vi "SingleJointedArmSim_example.vi"() -> ()   [LabVIEW 2019]
uses:
  <vilib>/Rock Robotics/WPI/ThirdParty/JAS_Junk/TrajLib/DCMOTOR.CTL
  <vilib>/Rock Robotics/WPI/ThirdParty/JAS_Junk/TrajLib/LINEAR_SYSTEM.ctl
  <vilib>/Analysis/Matrix/Datatypes/RealMatrix.ctl
  <vilib>/Rock Robotics/WPI/ThirdParty/JAS_Junk/TrajLib/LINEAR_QUADRATIC_REGULATOR.ctl
  <vilib>/Rock Robotics/WPI/ThirdParty/JAS_Junk/TrajLib/KALMAN_FILTER.ctl
  <vilib>/Rock Robotics/WPI/ThirdParty/JAS_Junk/TrajLib/LINEAR_SYSTEM_LOOP.ctl
  <vilib>/Rock Robotics/WPI/ThirdParty/JAS_Junk/TrajLib/LINEAR_PLANT_INV_FF.ctl
  <vilib>/Rock Robotics/WPI/ThirdParty/JAS_Junk/TrajLib/SINGLE_JOINT_ARM_SIM.ctl
  <vilib>/Rock Robotics/WPI/ThirdParty/JAS_Junk/TrajLib/LINEAR_SYSTEM_SIM.ctl
  <vilib>/Rock Robotics/WPI/ThirdParty/JAS_Junk/TrajLib/MatBuilder_Create.vi
  <vilib>/Rock Robotics/WPI/ThirdParty/JAS_Junk/TrajLib/DCMotor_New.vi
  <vilib>/Rock Robotics/WPI/ThirdParty/JAS_Junk/TrajLib/Units_RotationsPerMinuteToRadiansPerSecond.vi
  <vilib>/Rock Robotics/WPI/ThirdParty/JAS_Junk/TrajLib/LinearSystem_New.vi
  <vilib>/Rock Robotics/WPI/ThirdParty/JAS_Junk/TrajLib/MatrixHelper_Zero.vi
  <vilib>/Rock Robotics/WPI/ThirdParty/JAS_Junk/TrajLib/MatBuilder_Fill.vi
  <vilib>/Rock Robotics/WPI/ThirdParty/JAS_Junk/TrajLib/MatrixHelper_CoerceSize.vi
  <vilib>/Rock Robotics/WPI/ThirdParty/JAS_Junk/TrajLib/Trajectory_Library.lvlib
  <vilib>/Analysis/Matrix/NI_Matrix.lvlib
panel:
  in  "Tab Control":T1(tab)
  out "Battery Voltage":dbl format="%20.3f"
  out "CO Chart":cluster{dbl, "Voltage":dbl}(graph)
  in  "Move Arm":bool
  out "Arm Position\nRadians":dbl(slide) scale=-1.0..4.0
  out "Arm Angle":dbl format="%20.3f"
  out "Cor Err":bool
  out "Kalman Filtered\nArm Angle":dbl format="%20.3f"
  out "PV Chart":T2(graph)
  out "Predict Err":bool
  out "Motor Volt Dmd (CO)":dbl format="%20.3f"
  out "At Top":bool
  out "At Bottom":bool
  out "Motor Amps":dbl format="%20.3f"
  out "Arm Motor":T3 {"Jr_KgM2" format="%13.5p"; "L_H" format="%13.5p"; "Kt_NMPerAmp" format="%13.5p"; "KvINV_RadPerSecPerVolt" format="%13.5p"; "R_Ohms" format="%13.5p"; "FreeSpeed_RadPerSec" format="%13.5p"; "FreeCurrent_Amps" format="%13.5p"; "StallCurrent_Amps" format="%13.5p"; "StallTorque_NM" format="%13.5p"; "nominalVoltage_Volts" format="%13.5p"}
  out "m_Arm":T4
  out "Single Joint Arm Simulaation":T6 {"GearBox"."Jr_KgM2" format="%13.5p"; "GearBox"."L_H" format="%13.5p"; "GearBox"."Kt_NMPerAmp" format="%13.5p"; "GearBox"."KvINV_RadPerSecPerVolt" format="%13.5p"; "GearBox"."R_Ohms" format="%13.5p"; "GearBox"."FreeSpeed_RadPerSec" format="%13.5p"; "GearBox"."FreeCurrent_Amps" format="%13.5p"; "GearBox"."StallCurrent_Amps" format="%13.5p"; "GearBox"."StallTorque_NM" format="%13.5p"; "GearBox"."nominalVoltage_Volts" format="%13.5p"}
  out "KalmanFilter":T8
  out "Kalman Error":errorcluster
  out "LinearQuadraticRegulator":T9
  out "LQR Error":bool
  out "Linear System Loop":T10
  out "LinSysLoop_Error":bool
  # "<States,States>"
  # "<States,Inputs>"
  # "<Outputs,States>"
  # "<Outputs,Inputs>"
  # "<States, 1>"
  # "<Outputs, 1>"
  # "<Inputs, 1>"
  # "<Outputs, 1>"
  # "<States,States>"
  # "<States,Inputs>"
  # "<Outputs,States>"
  # "<Outputs,Inputs>"
  # "Steady State Gain  \n<States,Outputs>"
  # "State Estimate <Statess,1>"
  # "<States,States>"
  # "<States,Inputs>"
  # "<Outputs,States>"
  # "<Outputs,Inputs>"
  # "Ref State <States,1>"
  # "Comp and capped \noutput <Inputs,1>"
  # "Controller gain\n<Inputs,States>"
  # "<States,1>"
  # "<FUTURE --- CLAMP TYPE -- For now\nuse Normalize>"
  # "Steady State Gain  \n<States,Outputs>"
  # "State Estimate <Statess,1>"
  # "<States,States>"
  # "<States,Inputs>"
  # "<Outputs,States>"
  # "<Outputs,Inputs>"
  # "<States,1>"
  # "<Inputs,1>"
  # "<States,Inputs>"
  # "<States,States>"
  # "Ref State <States,1>"
  # "Comp and capped \noutput <Inputs,1>"
  # "Controller gain\n<Inputs,States>"
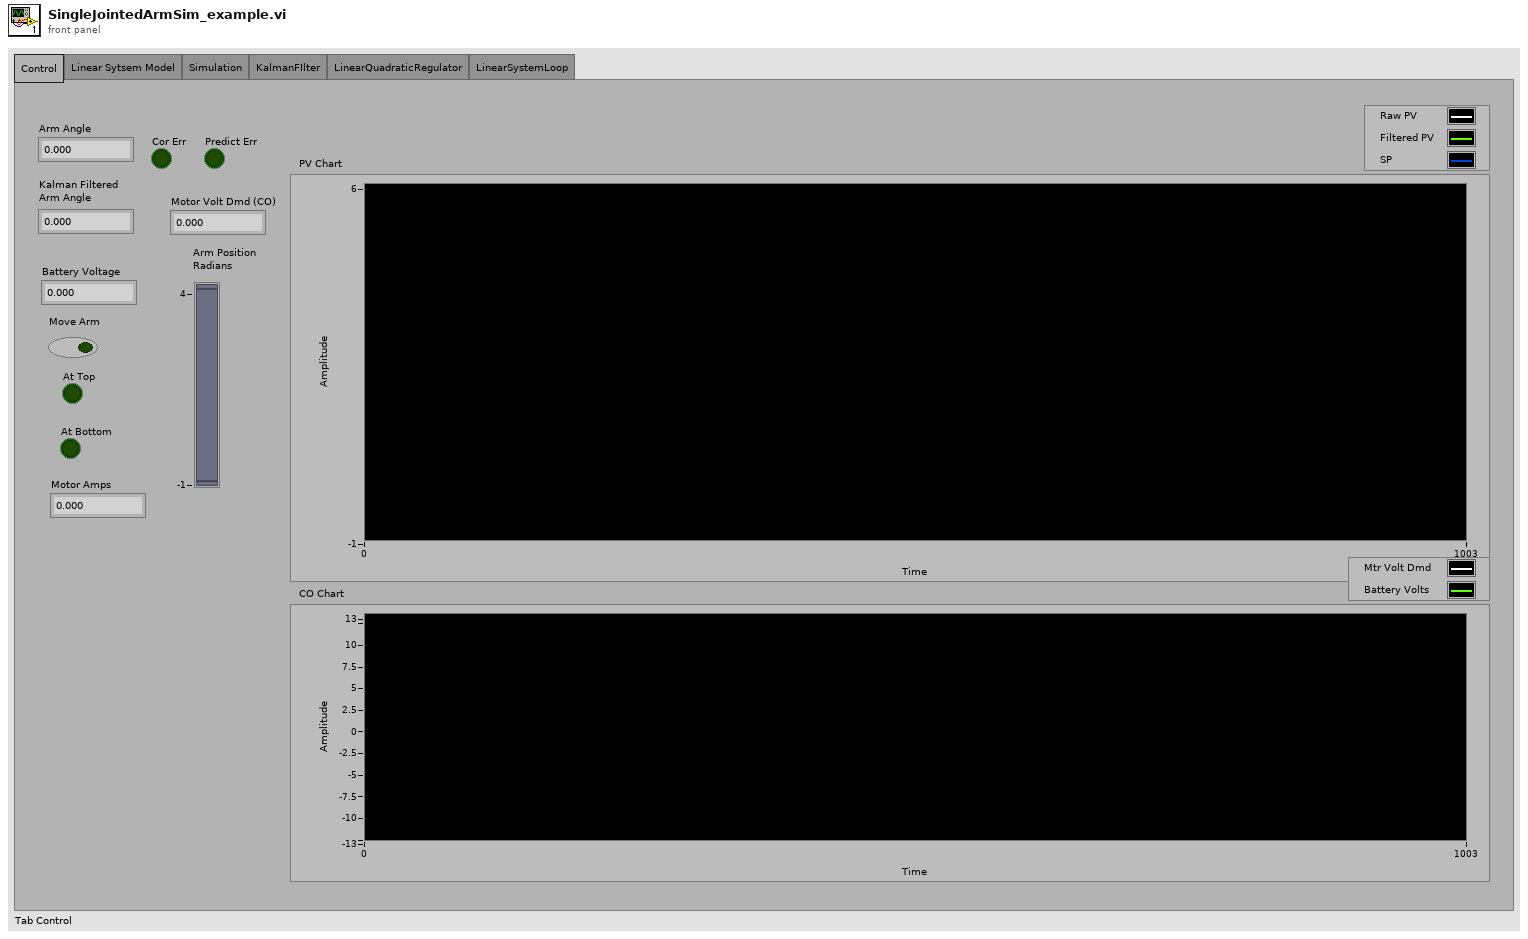
[diagram p1: front panel]
types:
  T1 = enum32{"Control", "Linear Sytsem Model", "Simulation", "KalmanFIlter", "LinearQuadraticRegulator", "LinearSystemLoop"}
  T2 = cluster{"upper limit":dbl, "Real Matrix Element":dbl, "Real Matrix Element":dbl}
  T3 = typedef "Trajectory_Library.lvlib/DCMOTOR.CTL" = cluster{"nominalVoltage_Volts":dbl, "StallTorque_NM":dbl, "StallCurrent_Amps":dbl, "FreeCurrent_Amps":dbl, "FreeSpeed_RadPerSec":dbl, "R_Ohms":dbl, "KvINV_RadPerSecPerVolt":dbl, "Kt_NMPerAmp":dbl, "L_H":dbl, "Jr_KgM2":dbl}
  T4 = typedef "Trajectory_Library.lvlib/LINEAR_SYSTEM.ctl" = cluster{"m_A":T5, "m_B":T5, "m_C":T5, "m_D":T5, "States":i32, "Inputs":i32, "Outputs":i32}
  T5 = typedef "NI_Matrix.lvlib/RealMatrix.ctl" = dbl[][]
  T6 = typedef "Trajectory_Library.lvlib/SINGLE_JOINT_ARM_SIM.ctl" = cluster{"Arm_LinearSystem":T7, "GearBox":T3, "Gearing":dbl, "R_ArmLength_M":dbl, "MinAngle_Rad":dbl, "MaxAngle_Rad":dbl, "ArmMass_Kg":dbl, "SimulateGravity":bool}
  T7 = typedef "Trajectory_Library.lvlib/LINEAR_SYSTEM_SIM.ctl" = cluster{"m_Plant":T4, "m_X":T5, "m_Y":T5, "m_U":T5, "MeasureStdDev":T5}
  T8 = typedef "Trajectory_Library.lvlib/KALMAN_FILTER.ctl" = cluster{"m_K":T5, "m_xHat":T5, "States":i32, "Outputs":i32, "m_Plant":T4}
  T9 = typedef "Trajectory_Library.lvlib/LINEAR_QUADRATIC_REGULATOR.ctl" = cluster{"m_r":T5, "m_U":T5, "m_K":T5, "States":i32, "Inputs":i32}
  T10 = typedef "Trajectory_Library.lvlib/LINEAR_SYSTEM_LOOP.ctl" = cluster{"Controller":T9, "FeedForward":T11, "Observer":T8, "Next_R":T5, "Clamp Max":T5}
  T11 = typedef "Trajectory_Library.lvlib/LINEAR_PLANT_INV_FF.ctl" = cluster{"m_R":T5, "m_Uff":T5, "m_B":T5, "m_A":T5, "States":i32, "Inputs":i32}
  T12 = cluster{"ArmAngle_Rad":dbl, "Real Matrix Element":dbl, "Real Matrix Element":dbl}
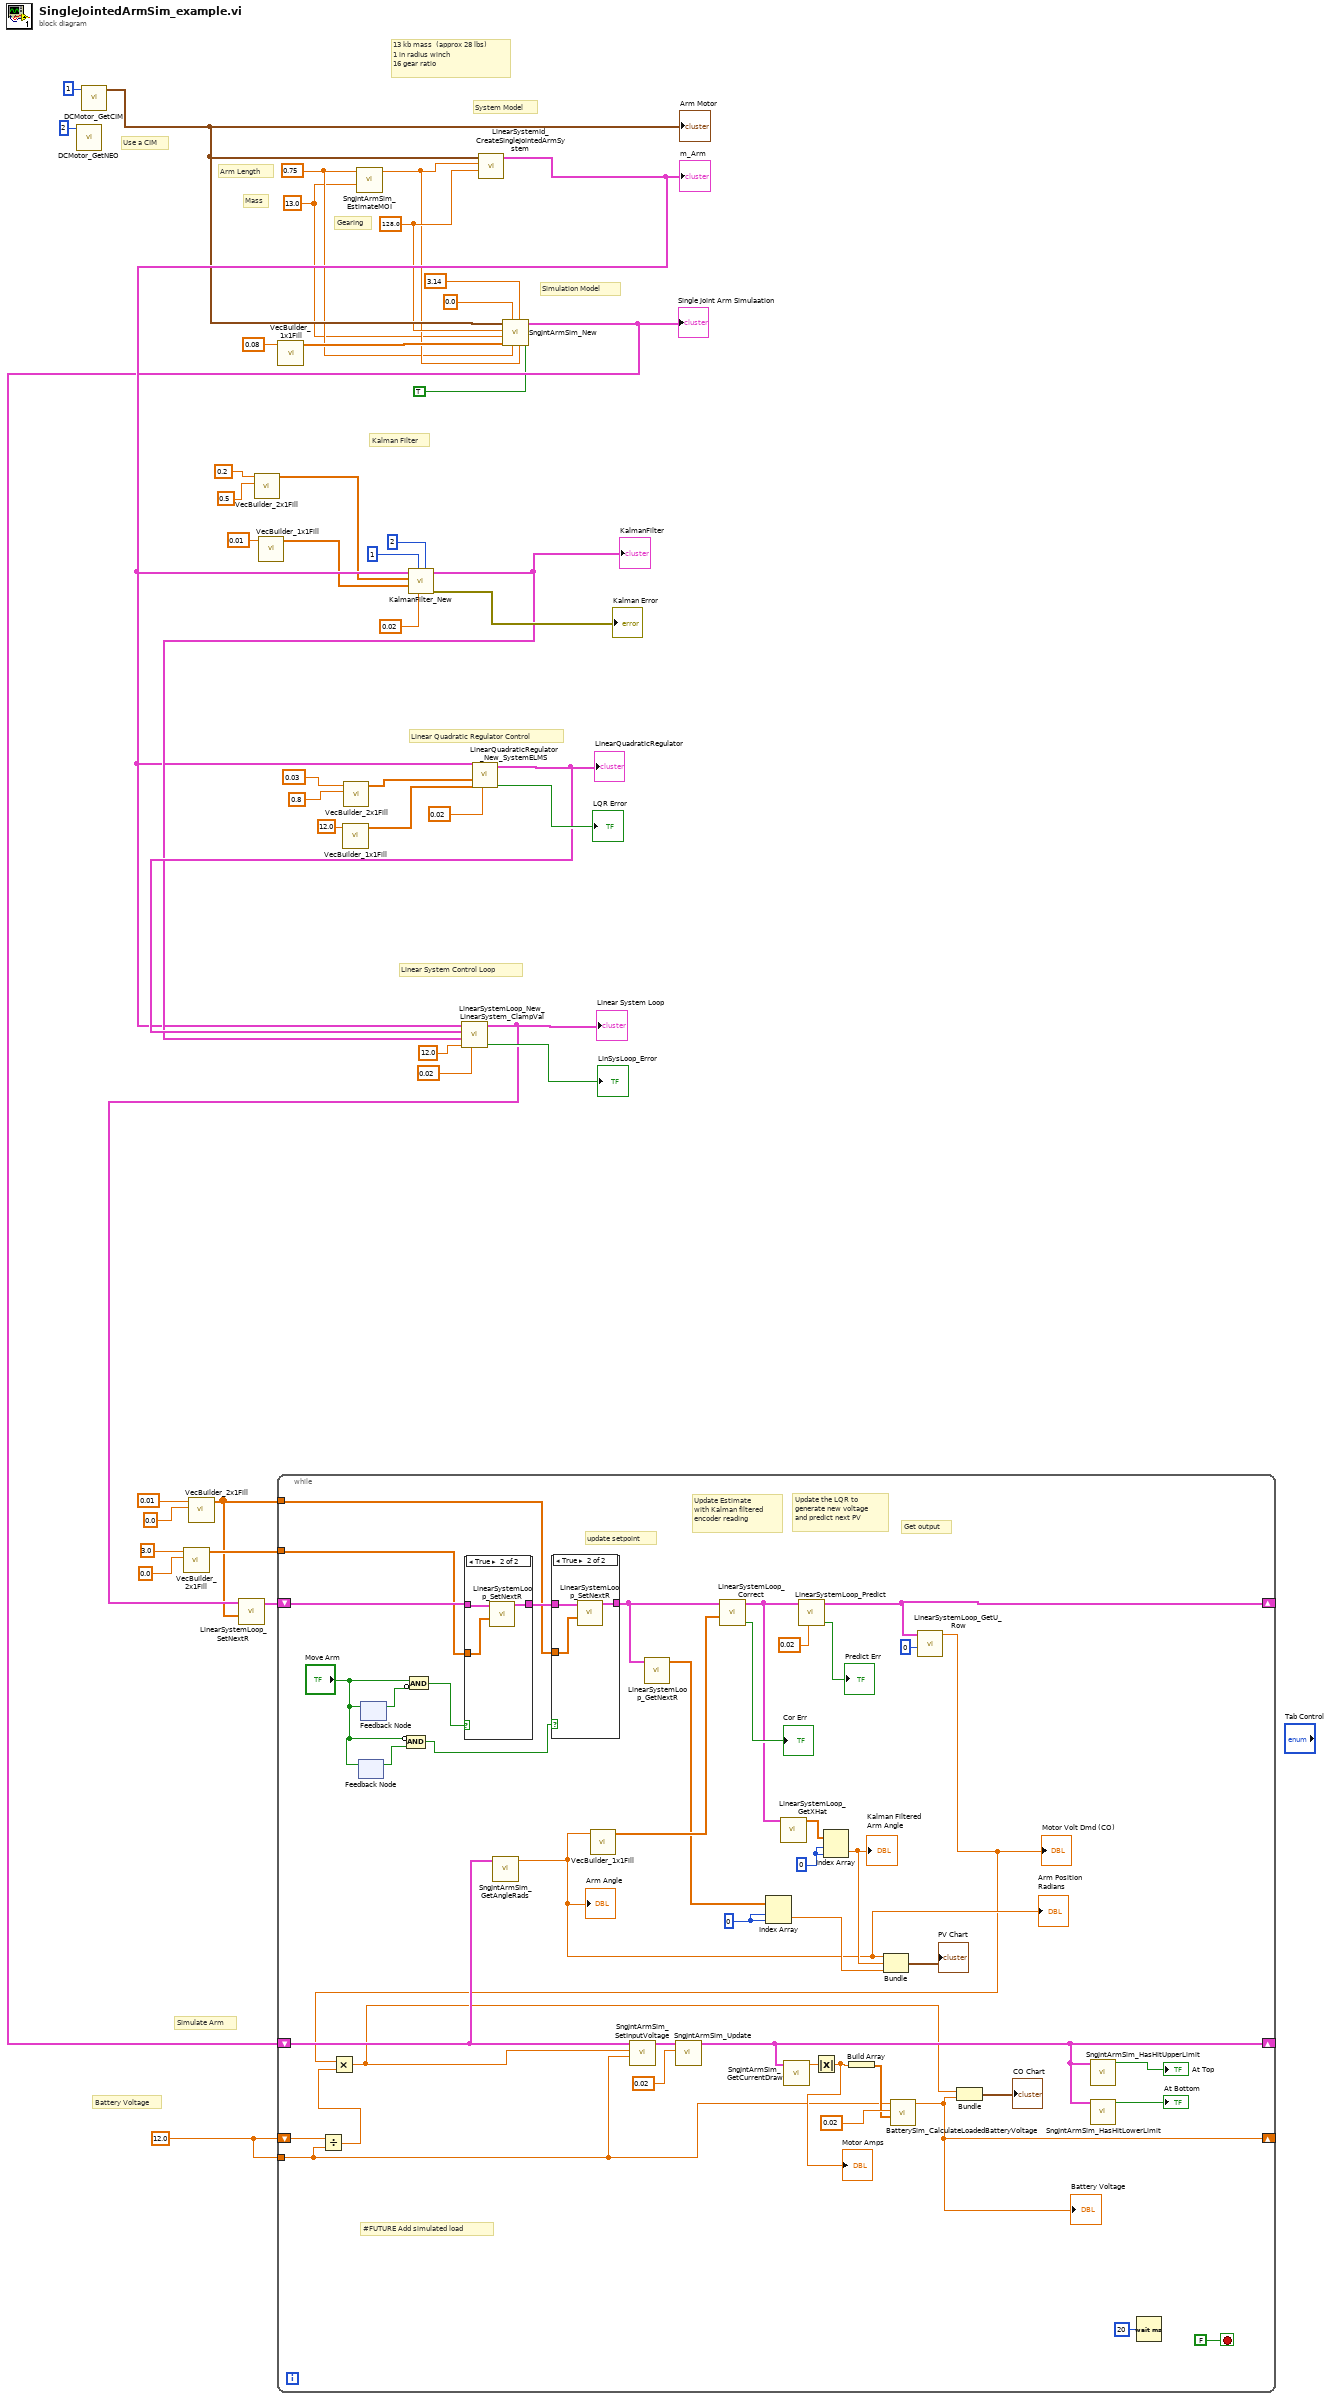
[diagram p0: block diagram]
diagram:
  w4 = 0.75 ("ArmLength_M")
  w7 = 128.0 ("G")
  w3 = 13.0 ("massKg")
  w36 = 12.0
  # "Simulation Model"
  # "System Model"
  # "Arm Length"
  # "Mass"
  # "Kalman Filter"
  # "Linear Quadratic Regulator Control"
  # "Linear System Control Loop"
  # "Simulate Arm"
  # "13 kb mass  (approx 28 lbs)\n1 in radius winch\n16 gear ratio"
  # "Gearing"
  # "Use a CIM"
  # "Battery Voltage"
  n1 = call <vilib>:"DCMotor_GetNEO.vi"("Num Motors"=2) -> ()  [unwired: 10 in, 1 out]
  n2 = call <vilib>:"DCMotor_GetCIM.vi"("Num Motors"=1) -> ("DCMOTOR"=w10:T3)  [unwired: 10 in]
  "Arm Motor" <- w10
  n3 = call <vilib>:"VecBuilder_2x1Fill.vi"("R1"=0.0, "R0"=3.0 ("RotationsPerMinute")) -> ("output matrix"=w16:T5)  [unwired: 9 in]
  n4 = call <vilib>:"VecBuilder_2x1Fill.vi"("R1"=0.0, "R0"=0.01 ("R0_C0")) -> ("output matrix"=w1:T5)  [unwired: 9 in]
  n5 = call <vilib>:"VecBuilder_2x1Fill.vi"("R1"=0.5, "R0"=0.2 ("R0_C0")) -> ("output matrix"=w27:T5)  [unwired: 9 in]
  n6 = call <vilib>:"VecBuilder_1x1Fill.vi"("R0_C0"=0.01) -> ("output matrix"=w26:T5)  [unwired: 10 in]
  n7 = call <vilib>:"VecBuilder_1x1Fill.vi"("R0_C0"=0.08) -> ("output matrix"=w6:T5)  [unwired: 10 in]
  n8 = call <vilib>:"VecBuilder_1x1Fill.vi"("R0_C0"=12.0) -> ("output matrix"=w20:T5)  [unwired: 10 in]
  n9 = call <vilib>:"VecBuilder_2x1Fill.vi"("R1"=0.8 ("R0_C0"), "R0"=0.03 ("R0_C0")) -> ("output matrix"=w22:T5)  [unwired: 9 in]
  n10 = call <vilib>:"SngJntArmSim_EstimateMOI.vi"("ArmMass_Kg"=w3, "ArmLength_M"=w4) -> ("MOI"=w5:dbl)  [unwired: 9 in]
  n11 = call <vilib>:"LinearSystemId_CreateSingleJointedArmSystem.vi"("G"=w7, "jKgSquaredMeters"=w5, "DCMOTOR"=w10) -> ("Linearsystem"=w34:T4)  [unwired: 7 in, 1 out]
  "m_Arm" <- w34
  n12 = call <vilib>:"KalmanFilter_New.vi"("States"=2, "dt_Seconds"=0.02, "Outputs"=1, "MeasurementStdDevs"=w26, "StateStdDevs"=w27, "Plant"=w34) -> ("Error"=→"Kalman Error":errorcluster, "KalmanFilter"=w40:T8)  [unwired: 4 in]
  "KalmanFilter" <- w40
  n13 = call <vilib>:"LinearQuadraticRegulator_New_SystemELMS.vi"("dt_Seconds"=0.02, "Relms"=w20, "Qelms"=w22, "LINEARSYSTEM"=w34) -> ("Error"=→"LQR Error":bool, "LinearQuadraticRegulator"=w41:T9)  [unwired: 6 in]
  "LinearQuadraticRegulator" <- w41
  n14 = call <vilib>:"LinearSystemLoop_New_LinearSystem_ClampVal.vi"("dT_Seconds"=0.02, "Max_Voltage"=12.0, "Observer"=w40, "Controller"=w41, "Plant"=w34) -> ("Error"=→"LinSysLoop_Error":bool, "Linear System Loop"=w12:T10)  [unwired: 5 in]
  "Linear System Loop" <- w12
  n15 = call <vilib>:"LinearSystemLoop_SetNextR.vi"("R"=w1, "input inear System Loop"=w12) -> ("out Linear System Loop"=w13:T10)  [unwired: 8 in, 1 out]
  n16 = call <vilib>:"SngJntArmSim_New.vi"("SimulateGravity"=TRUE, "jKgMetersSquared"=w5, "MaxAngle_Rad"=3.14 ("MaxHeight_Meters"), "ArmLength_Meters"=w4, "MinAngle_Rad"=0.0 ("MinHeight_Meters"), "MeasurementStdDev"=w6, "ArmMass_Kg"=w3, "Gearing"=w7, "GearBox"=w10) -> ("SingleJointArmSim"=w11:T6)  [unwired: 1 in, 1 out]
  "Single Joint Arm Simulaation" <- w11
  n17 = while {
    shift-right: [w63] -> _
    shift-left: w13 -> [w56]
    tunnel: w16 -> [w54]
    tunnel: w1 -> [w55]
    shift-right: [w58] -> _
    shift-left: w11 -> [w48]
    shift-right: [w64] -> _
    shift-left: w36 -> [w69]
    tunnel: w36 -> [w46]
    stop <- FALSE stop-if-true
    w71 = 0 ("index (row)")
    w81 = 0 ("index (row)")
    # "#FUTURE Add simulated load"
    # "Get output"
    # "Update the LQR to \ngenerate new voltage\nand predict next PV"
    # "update setpoint"
    # "Update Estimate\nwith Kalman filtered\nencoder reading"
    n18 = Divide(x=w69, y=w46) -> (x/y=w68:dbl)
    n19 = feedback #1() -> (w85:bool)  [unwired: 1 in]
    n20 = feedback-in #1("Move Arm") -> ()
    n21 = feedback-in #2("Move Arm") -> ()
    n22 = feedback #2() -> (w86:bool)  [unwired: 1 in]
    n23 = Compound Arithmetic op=AND(invert "Move Arm", w85) -> (w52:bool)
    n24 = Compound Arithmetic op=AND("Move Arm", invert w86) -> (w53:bool)
    n25 = case shown="True" w53 {
      tunnel: [w89 w92] -> w57
      tunnel: w56 -> [w89 w91]
      tunnel: w54 -> [_ w90]
      frame False {
      }
      frame True {
        n26 = call <vilib>:"LinearSystemLoop_SetNextR.vi"("R"=w90, "input inear System Loop"=w91) -> ("out Linear System Loop"=w92:T10)  [unwired: 8 in, 1 out]
      }
    }
    n27 = call <vilib>:"SngJntArmSim_GetAngleRads.vi"("SingleJointArmSim"=w48) -> ("ArmAngle_Rad"=w49:dbl)  [unwired: 10 in]
    "Arm Position\nRadians" <- w49
    "Arm Angle" <- w49
    n28 = case shown="True" w52 {
      tunnel: [w93 w96] -> w51
      tunnel: w57 -> [w93 w95]
      tunnel: w55 -> [_ w94]
      frame False {
      }
      frame True {
        n29 = call <vilib>:"LinearSystemLoop_SetNextR.vi"("R"=w94, "input inear System Loop"=w95) -> ("out Linear System Loop"=w96:T10)  [unwired: 8 in, 1 out]
      }
    }
    n30 = call <vilib>:"VecBuilder_1x1Fill.vi"("R0_C0"=w49) -> ("output matrix"=w83:T5)  [unwired: 10 in]
    n31 = call <vilib>:"LinearSystemLoop_GetNextR.vi"("input inear System Loop"=w51) -> ("NextR"=w50:T5)  [unwired: 10 in]
    n32 = call <vilib>:"LinearSystemLoop_Correct.vi"("Y"=w83, "input inear System Loop"=w51) -> ("Error"=→"Cor Err":bool, "out Linear System Loop"=w77:T10)  [unwired: 8 in]
    n33 = Index Array(array=w50, index (row)=w71, index (col)=w71) -> (element=w70:dbl)
    n34 = call <vilib>:"LinearSystemLoop_GetXHat.vi"("input inear System Loop"=w77) -> ("XHat"=w80:T5)  [unwired: 10 in]
    n35 = call <vilib>:"LinearSystemLoop_Predict.vi"("dT_Seconds"=0.02, "input inear System Loop"=w77) -> ("Error"=→"Predict Err":bool, "out Linear System Loop"=w63:T10)  [unwired: 8 in]
    n36 = Index Array(array=w80, index (row)=w81, index (col)=w81) -> (element=w79:dbl)
    "Kalman Filtered\nArm Angle" <- w79
    n37 = Bundle("ArmAngle_Rad"=w49, "Real Matrix Element"=w79, "Real Matrix Element"=w70) -> (→"PV Chart":T12)  [unwired: 1 in]
    n38 = call <vilib>:"LinearSystemLoop_GetU_Row.vi"("Row"=0, "input inear System Loop"=w63) -> ("U"=w47:dbl)  [unwired: 9 in]
    "Motor Volt Dmd (CO)" <- w47
    n39 = Multiply(x=w47, y=w68) -> (x*y=w45:dbl)
    n40 = call <vilib>:"SngJntArmSim_SetInputVoltage.vi"("Battery_Volts"=w46, "Input_Voltage"=w45, "in SingleJointArmSim"=w48) -> ("out SingleJointArmSim"=w73:T6)  [unwired: 8 in]
    n41 = call <vilib>:"SngJntArmSim_Update.vi"("dT_Seconds"=0.02, "in SingleJointArmSim"=w73) -> ("out SingleJointArmSim"=w58:T6)  [unwired: 8 in, 1 out]
    n42 = call <vilib>:"SngJntArmSim_GetCurrentDraw.vi"("SingleJointArmSim"=w58) -> ("Current_Amps"=w60:dbl)  [unwired: 10 in]
    n43 = Absolute Value(x=w60) -> (abs(x)=w59:dbl)
    "Motor Amps" <- w59
    n44 = Build Array(w59) -> (w66:dbl[])
    n45 = call <vilib>:"BatterySim_CalculateLoadedBatteryVoltage.vi"("Currents"=w66, "Resistance_Ohms"=0.02, "NominalVoltage"=w46) -> ("Voltage"=w64:dbl)  [unwired: 8 in]
    "Battery Voltage" <- w64
    n46 = Bundle(w45, "Voltage"=w64) -> (→"CO Chart":cluster{dbl, "Voltage":dbl})  [unwired: 1 in]
    n47 = call <vilib>:"SngJntArmSim_HasHitUpperLimit.vi"("SingleJointArmSim"=w58) -> ("At HIgh LImit"=→"At Top":bool)  [unwired: 10 in]
    n48 = call <vilib>:"SngJntArmSim_HasHitLowerLimit.vi"("SingleJointArmSim"=w58) -> ("AtLowLimit"=→"At Bottom":bool)  [unwired: 10 in]
    n49 = Wait (ms)(milliseconds to wait=u32 20) -> ()  [unwired: 1 out]
  }
